vi "Live Button Off.vi"(8 "error in (no error)":errorcluster, 11 "Main Window in":refnum<class "Main Window.lvclass">) -> (0 "error out":errorcluster, 3 "Main Window out":refnum<class "Main Window.lvclass">)   [LabVIEW 2015, in "Main Window.lvlib" / "Main Window.lvclass"]
uses:
  Main Window.lvclass
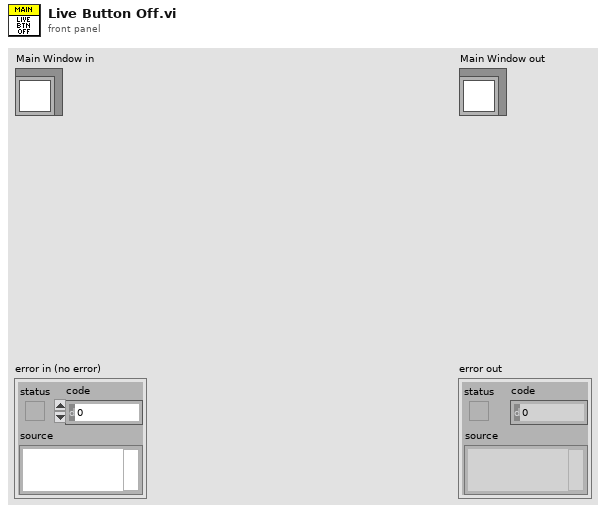
[diagram p1: front panel]
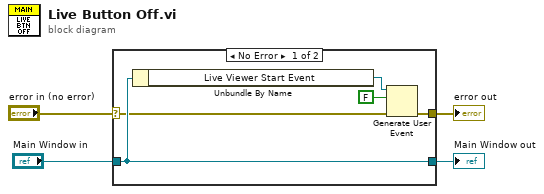
[diagram p0: block diagram]
diagram:
  n1 = case shown="No Error" "error in (no error)" {
    selector: "error in (no error)" -> [w5 w11]
    tunnel: [w7 w11] -> w3
    tunnel: [w6 w10] -> w1
    tunnel: "Main Window in" -> [w6 w10]
    frame No Error {
      n2 = Unbundle By Name(w6) -> ("Live Viewer Start Event"=w9:refnum<user-event>)
      n3 = Generate User Event(user event=w9, event data cluster=FALSE ("event data"), error in=w5) -> (error out=w7:errorcluster)  [unwired: 1 in, 1 out]
    }
    frame Error {
    }
  }
  "error out" <- w3
  "Main Window out" <- w1
